vi "Display Results.vi"(8 "Error In":errorcluster, 11 "Pass":bool) -> (0 "Error Out":errorcluster)   [LabVIEW 2021]
doc: "Displays the outcome (Error, Pass/Fail)."
uses:
  <vilib>/picture/picture.llb/imagedata.ctl
panel:
  out "Details":string
  out "Resolution":string
  in  "Ok":bool
  out "picture":picture
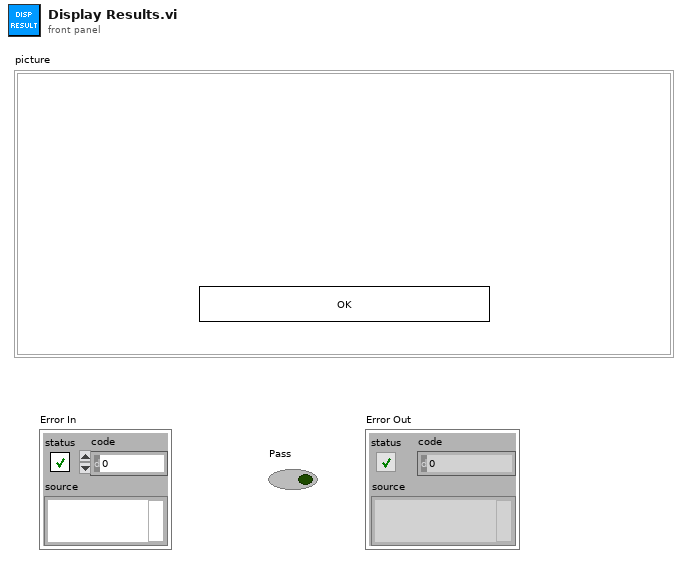
[diagram p1: front panel]
types:
  T1 = typedef "imagedata.ctl" = cluster{"image type":i32, "image depth":i32, "image":u8[], "mask":u8[], "colors":u32[], "Rectangle":cluster{"left":i16, "top":i16, "right":i16, "bottom":i16}}
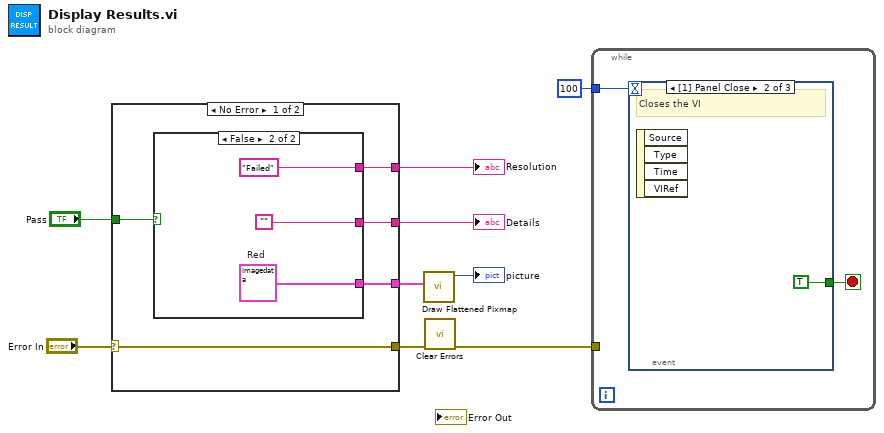
[diagram p0: block diagram]
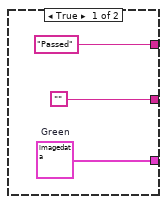
[diagram p2: hidden frame]
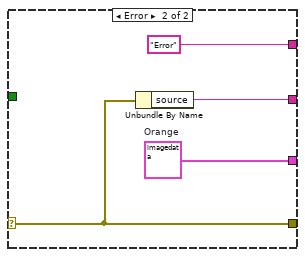
[diagram p3: hidden frame]
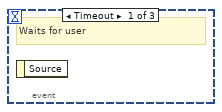
[diagram p4: hidden frame]
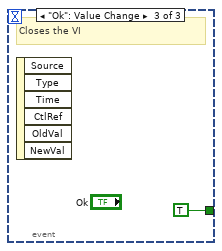
[diagram p5: hidden frame]
diagram:
  n1 = case shown="No Error" "Error In" {
    selector: "Error In" -> [w14 w23]
    tunnel: [w14 w23] -> w2
    tunnel: [w12 w24] -> w7
    tunnel: [w10 w22] -> w5
    tunnel: [w11 "Error" ("Resolution")] -> w4
    tunnel: "Pass" -> [w13 _]
    frame No Error {
      n2 = case shown="False" w13 {
        tunnel: [w17 w18] -> w12
        tunnel: ["Passed" "Failed"] -> w11
        tunnel: ["" ""] -> w10
        frame True {
          w17 = T1 {"image type"=0, "image depth"=24, "image"=array[586380 elements], "mask"=[], "colors"=[], "Rectangle"={"left"=0, "top"=0, "right"=674, "bottom"=290}}  # Green
        }
        frame False {
          w18 = T1 {"image type"=0, "image depth"=24, "image"=array[586380 elements], "mask"=[], "colors"=[], "Rectangle"={"left"=0, "top"=0, "right"=674, "bottom"=290}}  # Red
        }
      }
    }
    frame Error {
      w24 = T1 {"image type"=0, "image depth"=24, "image"=array[586380 elements], "mask"=[], "colors"=[], "Rectangle"={"left"=0, "top"=0, "right"=674, "bottom"=290}}  # Orange
      n3 = Unbundle By Name(w23) -> ("source"=w22:string)
    }
  }
  "Resolution" <- w4
  "Details" <- w5
  n4 = call <vilib>:"Draw Flattened Pixmap.vi"("image data"=w7) -> ("new picture"=→"picture":picture)  [unwired: 8 in]
  n5 = call <vilib>:"Clear Errors.vi"("error in (no error)"=w2) -> ("error out"=w1:errorcluster)  [unwired: 5 in, 1 out]
  n6 = while {
    tunnel: 100 -> [w26]
    tunnel: w1 -> [_]
    stop <- w25 stop-if-true
    n7 = event shown="[1] Panel Close" {
      selector: _ -> [_ _ _]
      dyn-events: _ -> [_ _ _]
      timeout: w26 -> [_ _ _]
      tunnel: [_ TRUE TRUE] -> w25
      event Timeout {
        # "Waits for user"
        n8 = event-data() -> ()  [unwired: 1 in, 1 out]
      }
      event Panel Close {
        # "Closes the VI"
        n9 = event-data() -> ()  [unwired: 1 in, 4 out]
      }
      event "Ok": Value Change {
        # "Closes the VI"
        n10 = event-data() -> ()  [unwired: 1 in, 6 out]
      }
    }
  }
